vi "Update_Dust_Info.vi"() -> ()   [LabVIEW 2013]
doc: "Updates the dust_info and dust_info_small tables. For use in the Dust Lab, so anyone changing the source can update the database with the new source before going downstairs."
uses:
  Private/Controls/dust type.ctl
  Private/Controls/source_builders.ctl
  Private/Controls/dust_type_indicator.ctl
  <vilib>/Utility/miscctls.llb/LVPointTypeDef.ctl
panel:
  in  "error in (no error)":errorcluster
  out "error out":errorcluster
  in  "Exit":bool
  in  "Clear Errors":bool
  out "Dust Properties small":T1
  in  "Update dust info small":bool
  out "Dust Type small":T2 {"Batch" step=1; "Type" step=1; "Dust Source Builder:" items=["Keith Drake", "Nick Beaty", "Anthony Shu", "David James", "John Fontanese"]}
  out "Dust Properties":T1
  in  "Update dust info":bool
  out "Dust Type":T2 {"Batch" step=1; "Type" step=1; "Dust Source Builder:" items=["Keith Drake", "Nick Beaty", "Anthony Shu", "David James", "John Fontanese"]}
  # "Dust Information - Small"
  # "Dust Information - Big"
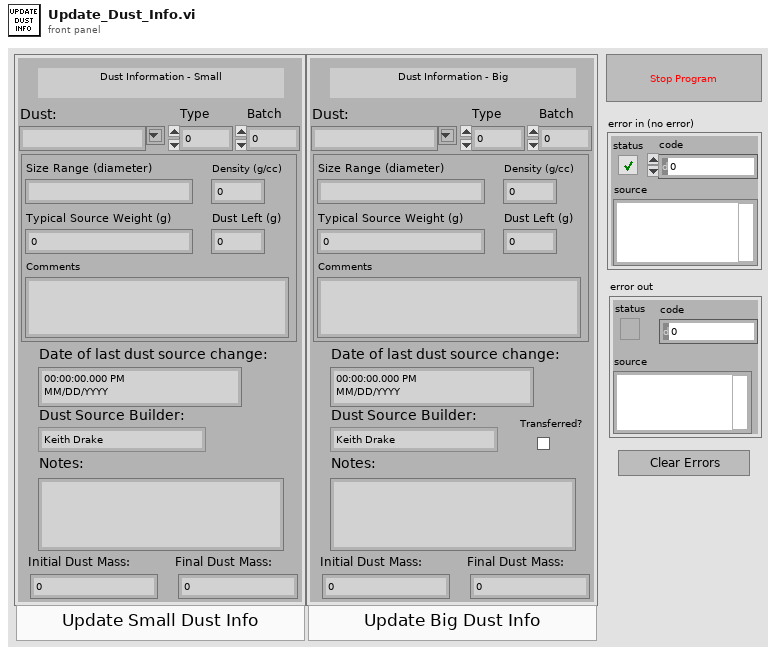
[diagram p1: front panel]
types:
  T1 = typedef "dust_type_indicator.ctl" = cluster{"Size Range (diameter)":string, "Density (g/cc)":dbl, "Typical Source Weight (g)":dbl, "Dust Left (g)":dbl, "Comments":string}
  T2 = typedef "dust type.ctl" = cluster{"Dust info id":u16, "Integer Timestamp":i64, "Dust:":string, "Dust Source Builder:":T3, "Notes:":string, "Date of last dust source change:":timestamp, "Initial Dust Mass:":dbl, "Final Dust Mass:":dbl, "Type":u16, "Batch":u16, "dust type id":u16, "Transferred?":bool}
  T3 = typedef "source_builders.ctl" = u16
  T4 = typedef "LVPointTypeDef.ctl" = cluster{"Horizontal":i16, "Vertical":i16}
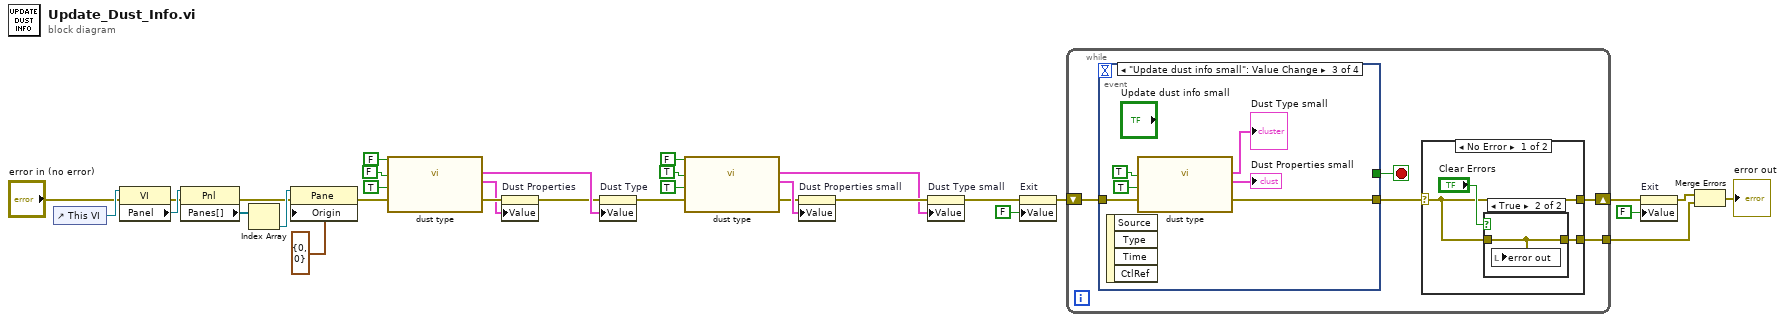
[diagram p0: block diagram]
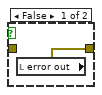
[diagram p2: hidden frame]
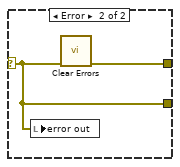
[diagram p3: hidden frame]
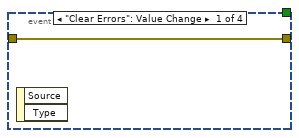
[diagram p4: hidden frame]
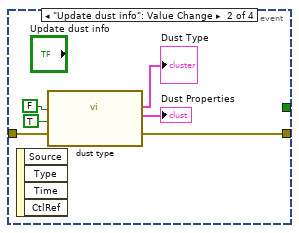
[diagram p5: hidden frame]
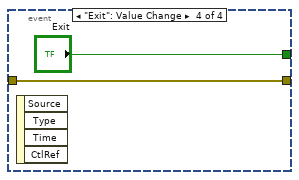
[diagram p6: hidden frame]
diagram:
  n1 = control-ref of="This VI"() -> (w25:refnum<vi>)
  n2 = property class="VI"(reference=w25, error in="error in (no error)") -> (error out=w26:errorcluster, "Panel"=w27:refnum<vi>)  [unwired: 1 out]
  n3 = property class="Pnl"(reference=w27, error in=w26) -> (error out=w28:errorcluster, "Panes[]"=w29:refnum<vi>[])  [unwired: 1 out]
  n4 = Index Array(array=w29) -> (element=w30:refnum<vi>)  [unwired: 1 in]
  n5 = property class="Pane"(reference=w30, error in=w28, "Origin"=T4 {"Horizontal"=0, "Vertical"=0}) -> (error out=w21:errorcluster)  [unwired: 1 out]
  n6 = call "dust type.vi"("Enable"=FALSE, "Small?"=FALSE, "Sub vi?"=TRUE, "error in (no error)"=w21) -> ("output cluster 2"=w19:T2, "Dust Properties 2"=w16:T1, "error out"=w17:errorcluster)  [unwired: 11 in, 2 out]
  n7 = property on="Dust Properties" class="Clust (strict)"(error in=w17, "Value"=w16) -> (error out=w18:errorcluster)  [unwired: 1 in, 1 out]
  n8 = property on="Dust Type" class="Clust (strict)"(error in=w18, "Value"=w19) -> (error out=w8:errorcluster)  [unwired: 1 in, 1 out]
  n9 = call "dust type.vi"("Enable"=FALSE, "Small?"=TRUE, "Sub vi?"=TRUE, "error in (no error)"=w8) -> ("output cluster 2"=w12:T2, "Dust Properties 2"=w15:T1, "error out"=w14:errorcluster)  [unwired: 11 in, 2 out]
  n10 = property on="Dust Properties small" class="Clust (strict)"(error in=w14, "Value"=w15) -> (error out=w13:errorcluster)  [unwired: 1 in, 1 out]
  n11 = property on="Dust Type small" class="Clust (strict)"(error in=w13, "Value"=w12) -> (error out=w6:errorcluster)  [unwired: 1 in, 1 out]
  n12 = property on="Exit" class="Bool (strict)"(error in=w6, "Value"=FALSE ("Exit")) -> (error out=w5:errorcluster)  [unwired: 1 in, 1 out]
  n13 = while {
    shift-right: [w35] -> w3
    shift-left: w5 -> [w33]
    tunnel: [w34] -> w32
    stop <- w37 stop-if-true
    n14 = event shown="[2] \"Update dust info small\": Value Change" {
      selector: _ -> [_ _ _ _]
      dyn-events: _ -> [_ _ _ _]
      timeout: _ -> [_ _ _ _]
      tunnel: w33 -> [w45 w50 w56 w58]
      tunnel: [w45 w51 w57 w58] -> w36
      tunnel: [_ _ _ "Exit"] -> w37
      event "Clear Errors": Value Change {
        n15 = event-data() -> ()  [unwired: 1 in, 2 out]
      }
      event "Update dust info": Value Change {
        n16 = event-data() -> ()  [unwired: 1 in, 4 out]
        n17 = call "dust type.vi"("Small?"=FALSE, "Sub vi?"=TRUE, "error in (no error)"=w50) -> ("output cluster 2"=→"Dust Type":T2, "Dust Properties 2"=→"Dust Properties":T1, "error out"=w51:errorcluster)  [unwired: 12 in, 2 out]
      }
      event "Update dust info small": Value Change {
        n18 = event-data() -> ()  [unwired: 1 in, 4 out]
        n19 = call "dust type.vi"("Small?"=TRUE, "Sub vi?"=TRUE, "error in (no error)"=w56) -> ("output cluster 2"=→"Dust Type small":T2, "Dust Properties 2"=→"Dust Properties small":T1, "error out"=w57:errorcluster)  [unwired: 12 in, 2 out]
      }
      event "Exit": Value Change {
        n20 = event-data() -> ()  [unwired: 1 in, 4 out]
      }
    }
    n21 = case shown="No Error" w36 {
      selector: w36 -> [w39 w43]
      tunnel: [w39 w44] -> w35
      tunnel: [w38 w43] -> w34
      frame No Error {
        n22 = case shown="True" "Clear Errors" {
          tunnel: w39 -> [_ w42]
          tunnel: [w41 w42] -> w38
          frame False {
            n23 = local read "error out"() -> (w41:errorcluster)
          }
          frame True {
            n24 = local write "error out"(w42) -> ()
          }
        }
      }
      frame Error {
        n25 = local write "error out"(w43) -> ()
        n26 = call <vilib>:"Clear Errors.vi"("error in (no error)"=w43) -> ("error out"=w44:errorcluster)  [unwired: 6 in]
      }
    }
  }
  n27 = property on="Exit" class="Bool (strict)"(error in=w3, "Value"=FALSE ("Exit")) -> (error out=w1:errorcluster)  [unwired: 1 in, 1 out]
  n28 = Merge Errors(w1, w32) -> (→"error out":errorcluster)
